vi "SQL_OpenIncidence.vi"(0 "ConnectionDSN":string, 1 "TableName":string, 2 "MachineName":string, 3 "StoppageReason":string, 4 "FolioEWO":string, 5 "FolioToolCrib":string) -> ()   [LabVIEW 2017]
panel:
  # "Insert into \"EPSL3\" values ('CW80','12:00','',80,'Electrodes Change','128654','45678','"
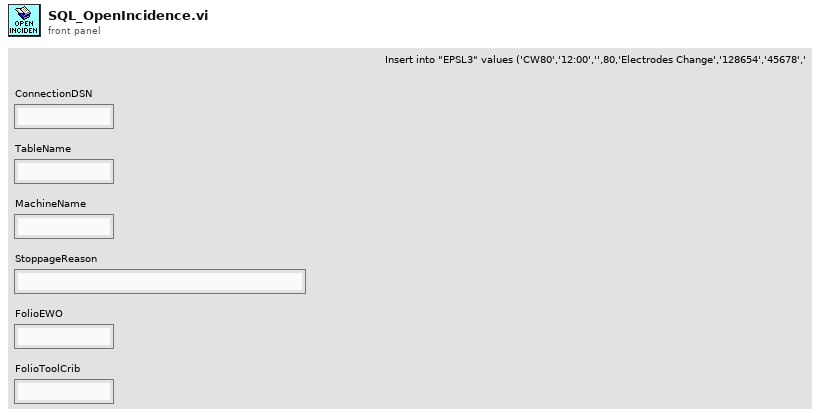
[diagram p1: front panel]
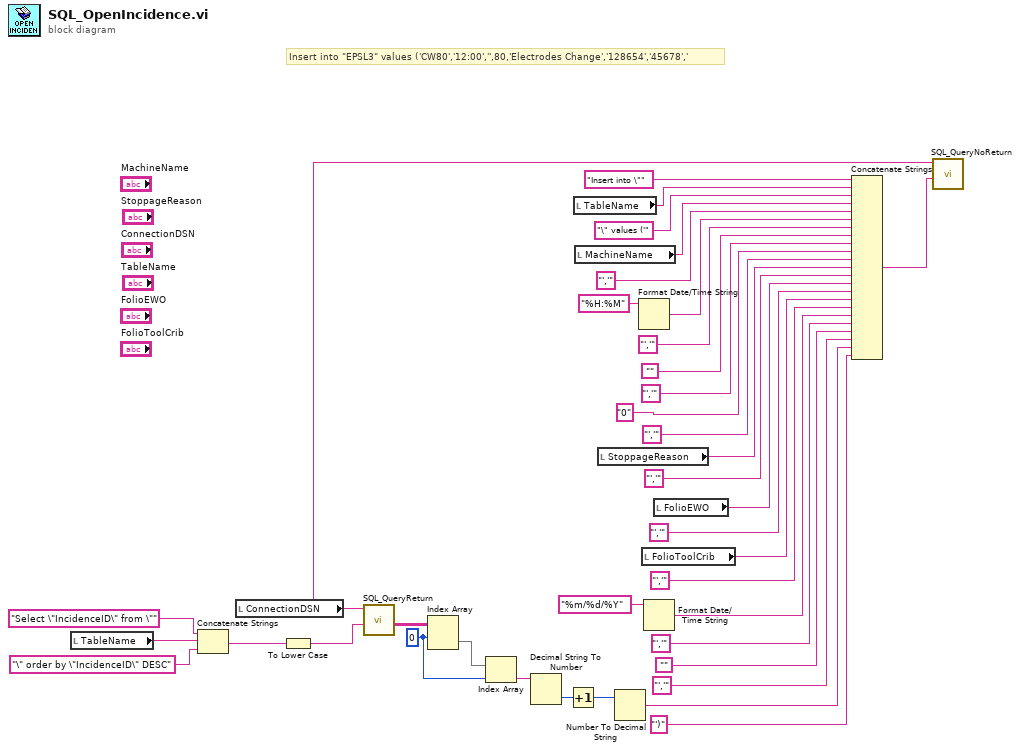
[diagram p0: block diagram]
diagram:
  w9 = 0 ("index (row)")
  # "Insert into \"EPSL3\" values ('CW80','12:00','',80,'Electrodes Change','128654','45678','"
  n1 = local read "TableName"() -> (w36:string)
  n2 = Concatenate Strings("Select \"IncidenceID\" from \"", w36, "\" order by \"IncidenceID\" DESC") -> (w7:string)
  n3 = local read "ConnectionDSN"() -> (w34:string)
  n4 = To Lower Case(string=w7) -> (all lower case string=w6:string)
  n5 = call "SQL_QueryReturn.vi"("SQL query"=w6, "ConnectionDSN"=w34) -> ("data"=w11:string[][])  [unwired: 9 in]
  n6 = Index Array(array=w11, index (row)=w9) -> (element=w10:string[])  [unwired: 1 in]
  n7 = Index Array(array=w10, index=w9) -> (element=w8:string)
  n8 = Decimal String To Number(string=w8) -> (number=w35:i32)  [unwired: 2 in, 1 out]
  n9 = Increment(x=w35) -> (x+1=w23:i32)
  n10 = local read "TableName"() -> (w32:string)
  n11 = local read "MachineName"() -> (w30:string)
  n12 = local read "StoppageReason"() -> (w20:string)
  n13 = Number To Decimal String(number=w23) -> (decimal integer string=w2:string)  [unwired: 1 in]
  n14 = Format Date/Time String(time format string (%c)="%H:%M") -> (date/time string=w27:string)  [unwired: 2 in]
  n15 = local read "FolioToolCrib"() -> (w16:string)
  n16 = Format Date/Time String(time format string (%c)="%m/%d/%Y") -> (date/time string=w12:string)  [unwired: 2 in]
  n17 = local read "FolioEWO"() -> (w18:string)
  n18 = Concatenate Strings("Insert into \"", w32, "\" values ('", w30, "','", w27, "','", "", "','", "0", "','", w20, "','", w18, "','", w16, "','", w12, "','", "", "','", w2, "')") -> (w22:string)
  n19 = call "SQL_QueryNoReturn.vi"("SQL query"=w22, "ConnectionDSN"=w34) -> ()  [unwired: 10 in]
